vi "Quench_CalcR(SubVI) 2.vi"(0 "Mag":fxp<+,16,14>, 5 "input valid":bool, 9 "count done?":bool) -> (4 "Tau meas":fxp<+/-,32,13>)   [LabVIEW 2025]
uses:
  <vilib>/rvi/FXPMathLib/FxpDiv/subVIs/nifxpmath_Div_SimConfig.ctl
  <vilib>/rvi/FXPMathLib/FxpDiv/simVIs/DllFxpDivTemp_sub.vi
  <vilib>/rvi/FXPMathLib/FxpSub/XNode/nifxpmath_Sub.xnode
  <vilib>/rvi/FXPMathLib/FxpInterpret/XNode/nifxpmath_Interpret.xnode
  <vilib>/rvi/FXPMathLib/FxpDiv/XNode/nifxpmath_Div.xnode
  <vilib>/rvi/FXPMathLib/sim/FxpSim.dll
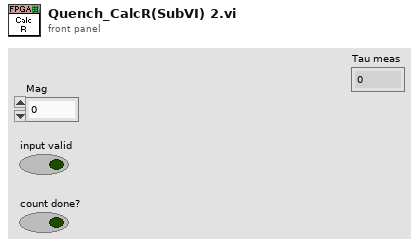
[diagram p1: front panel]
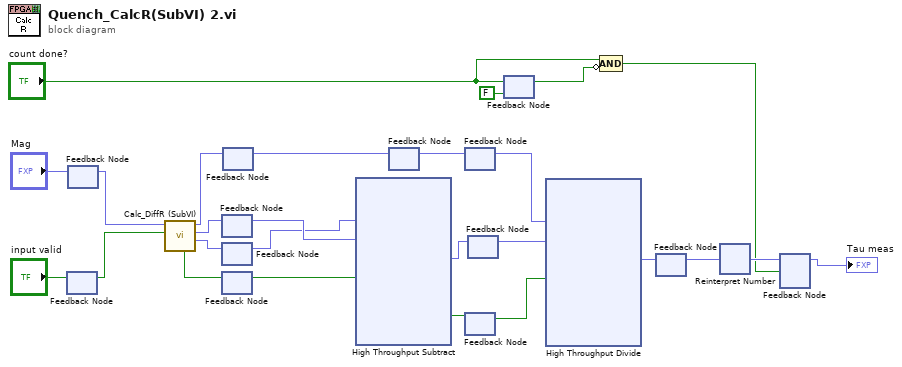
[diagram p0: block diagram]
diagram:
  n1 = feedback #1() -> (w19:bool)  [unwired: 1 in]
  n2 = feedback-in #1("input valid") -> ()
  n3 = feedback #2() -> (w18:fxp<+,16,14>)  [unwired: 1 in]
  n4 = feedback-in #2("Mag") -> ()
  n5 = call "Calc_DiffR (SubVI).vi"("input valid in"=w19, "Mag 3"=w18) -> ("Mag 1"=w15:fxp<+,16,14>, "Mag 2"=w16:fxp<+,16,14>, "Mag 4"=w17:fxp<+,16,14>, "input valid out"=w14:bool)  [unwired: 6 in]
  n6 = feedback #3() -> (w5:fxp<+,16,14>)  [unwired: 1 in]
  n7 = feedback-in #3(w16) -> ()
  n8 = feedback #4() -> (w4:fxp<+,16,14>)  [unwired: 1 in]
  n9 = feedback-in #4(w15) -> ()
  n10 = feedback #5() -> (w13:bool)  [unwired: 1 in]
  n11 = feedback-in #5(w14) -> ()
  n12 = feedback #6() -> (w12:fxp<+,16,14>)  [unwired: 1 in]
  n13 = feedback-in #6(w17) -> ()
  n14 = xnode "High Throughput Subtract"("x"=w4, "y"=w5, "input valid"=w13) -> ("x-y"=w11:fxp<+/-,16,14>, "output valid"=w25:bool)  [unwired: 1 in, 1 out]
  n15 = feedback #7() -> (w23:fxp<+,16,14>)  [unwired: 1 in]
  n16 = feedback-in #7(w12) -> ()
  n17 = feedback #8() -> (w7:fxp<+,16,14>)  [unwired: 1 in]
  n18 = feedback-in #8(w23) -> ()
  n19 = feedback #9() -> (w6:bool)  [unwired: 1 in]
  n20 = feedback-in #9(w25) -> ()
  n21 = feedback #10() -> (w8:fxp<+/-,16,14>)  [unwired: 1 in]
  n22 = feedback-in #10(w11) -> ()
  n23 = feedback #11(FALSE ("count done?")) -> (w22:bool)
  n24 = feedback-in #11("count done?") -> ()
  n25 = xnode "High Throughput Divide"("x"=w7, "y"=w8, "input valid"=w6) -> ("x/y"=w9:fxp<+/-,32,18>)  [unwired: 1 in, 2 out]
  n26 = Compound Arithmetic op=AND("count done?", invert w22) -> (w2:bool)
  n27 = feedback #12() -> (w10:fxp<+/-,32,18>)  [unwired: 1 in]
  n28 = feedback-in #12(w9) -> ()
  n29 = xnode "Reinterpret Number"("x"=w10) -> ("y"=w3:fxp<+/-,32,13>)
  n30 = feedback #13() -> (→"Tau meas":fxp<+/-,32,13>)  [unwired: 1 in]
  n31 = feedback-in #13(w3, w2) -> ()
